vi "Event Handler.vi"(8 "error in (no error)":errorcluster, 10 "Stop Event Handler":refnum<user-event>, 11 "D_Datagrid in":refnum<class "D_Datagrid.lvclass">) -> (0 "error out":errorcluster)   [LabVIEW 2023, in "D Datagrid Library.lvlib" / "D_Datagrid.lvclass"]
doc: "The <b>Event Handler VI</b> is a dynamic dispatch VI that should be overwritten if events are needed to create the enhanced QControl. \n\nBy inheriting from the main Control.lvclass the overwritten <b>Event Handler VI</b> will be launched asynchronously in the initialization of the QControl.\n<b> </b> <b> </b>\n©2016 Q Software Innovations, LLC (QSI)\nwritten by Quentin Alldredge\nproduced in LabVIEW 2015\n\nsupport@qsoftwareinnovations.com\nwww.qsoftwareinnovations.com\n\nAll rights reserved.\n\nRedistribution and use in source and binary forms, with or without modification, are permitted provided that the following conditions are met:\n\n * Redistributions of source code must retain the above copyright notice, this list of conditions and the following disclaimer.\n * Redistributions in binary form must reproduce the above copyright notice, this list of conditions and the following disclaimer in the documentation and/or other materials provided with the distribution.\n * Neither the name of Q Software Innovations, LLC. nor the names of its contributors may be used to endorse or promote products derived from this software without specific prior written permission.\n\nTHIS SOFTWARE IS PROVIDED BY THE COPYRIGHT HOLDERS AND CONTRIBUTORS \"AS IS\" AND ANY EXPRESS OR IMPLIED WARRANTIES, INCLUDING, BUT NOT LIMITED TO, THE IMPLIED WARRANTIES OF MERCHANTABILITY AND FITNESS FOR A PARTICULAR PURPOSE ARE DISCLAIMED. IN NO EVENT SHALL THE COPYRIGHT OWNER OR CONTRIBUTORS BE LIABLE FOR ANY DIRECT, INDIRECT, INCIDENTAL, SPECIAL, EXEMPLARY, OR CONSEQUENTIAL DAMAGES (INCLUDING, BUT NOT LIMITED TO, PROCUREMENT OF SUBSTITUTE GOODS OR SERVICES; LOSS OF USE, DATA, OR PROFITS; OR BUSINESS INTERRUPTION) HOWEVER CAUSED AND ON ANY THEORY OF LIABILITY, WHETHER IN CONTRACT, STRICT LIABILITY, OR TORT (INCLUDING NEGLIGENCE OR OTHERWISE) ARISING IN ANY WAY OUT OF THE USE OF THIS SOFTWARE, EVEN IF ADVISED OF THE POSSIBILITY OF SUCH DAMAGE."
uses:
  D_Datagrid.lvclass
  <vilib>/Utility/miscctls.llb/LVRowAndColumnTypeDef.ctl
  D_Datagrid.lvclass/D_Datagrid.ctl
  DatagridElement/DatagridElement.lvclass/DatagridElement.ctl
  DatagridElement/Read Enabled state.vi
  Read DataElements.vi
  Write DataElements.vi
  Read Auto update indicator.vi
  Redraw full indicator.vi
  <vilib>/Utility/cursorutil.llb/Set Cursor (Icon Pict).vi
  DatagridElement/DatagridElement.lvclass
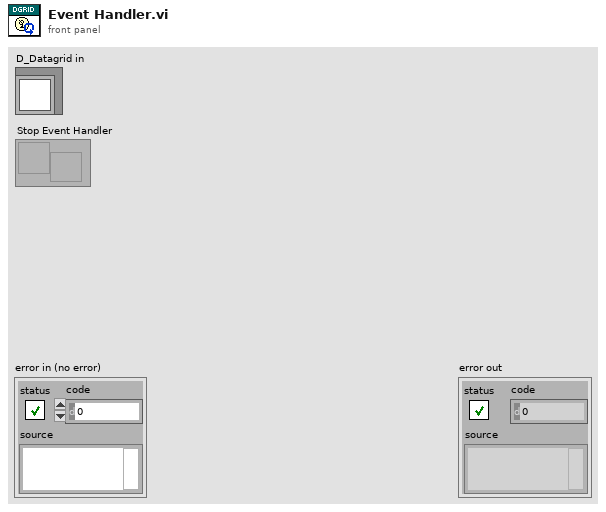
[diagram p1: front panel]
types:
  T1 = typedef "LVRowAndColumnTypeDef.ctl" = cluster{"Row":i32, "Column":i32}
  T2 = typedef "LVPoint32TypeDef.ctl" = cluster{"Horizontal":i32, "Vertical":i32}
  T3 = typedef "LVRectTypeDef.ctl" = cluster{"Left":i16, "Top":i16, "Right":i16, "Bottom":i16}
  T4 = enum8{"Enabled", "Disabled", "Disabled and Grayed Out"}
  T5 = typedef "D Datagrid Library.lvlib/D_Datagrid.lvclass/Scrolling behavior.ctl" = enum16{"Default", "Locked", "Displayed items only"}
  T6 = typedef "LVRowAndColumnUnsignedTypeDef.ctl" = cluster{"Row":u32, "Column":u32}
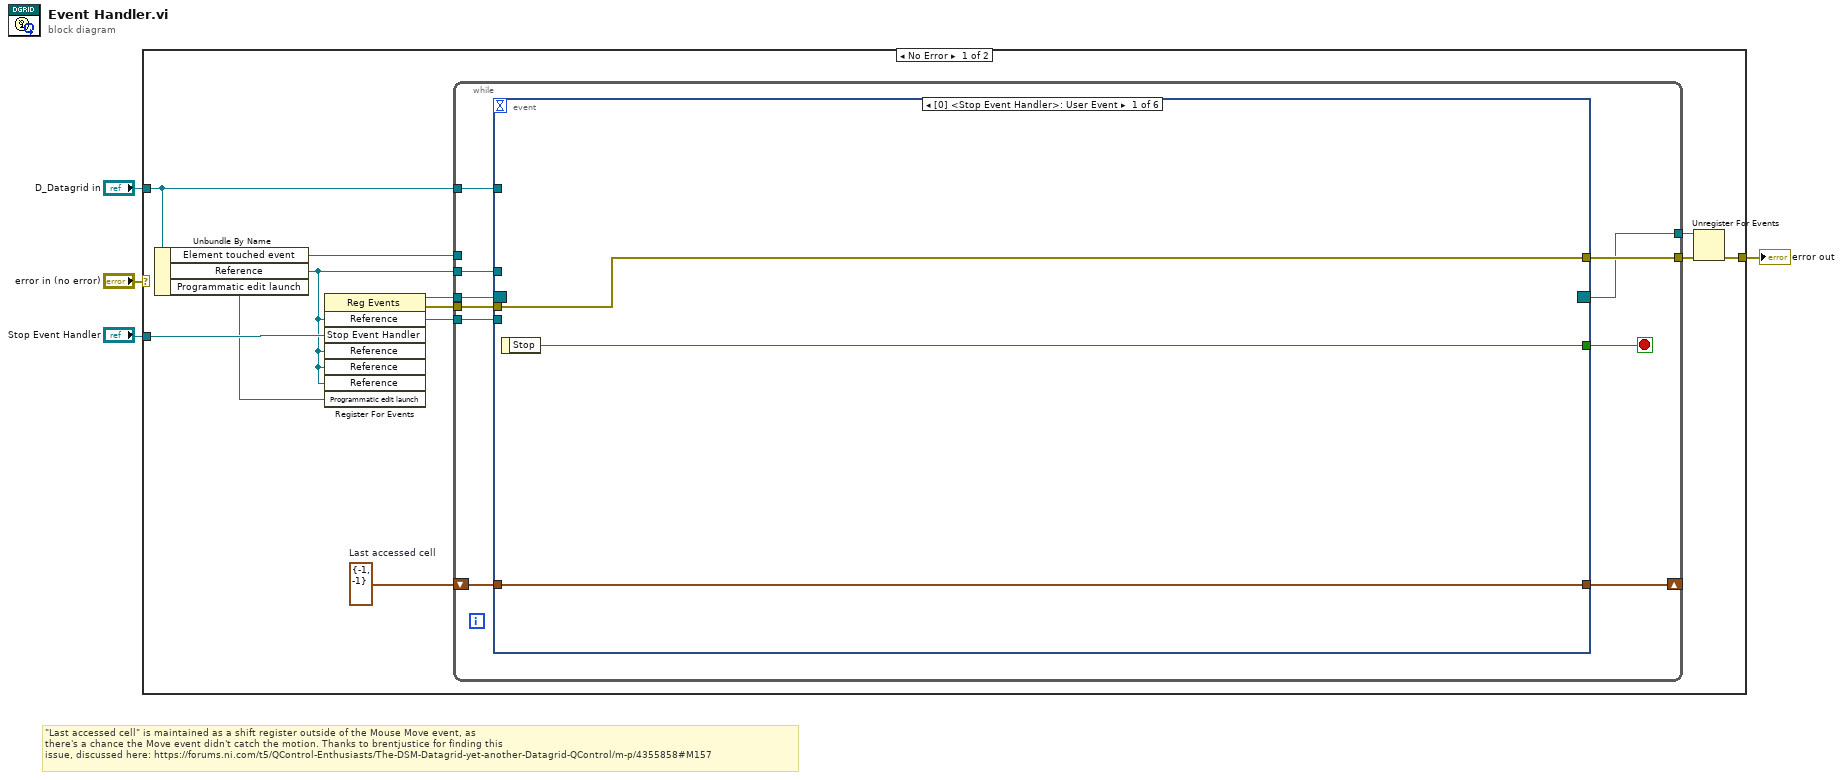
[diagram p0: block diagram]
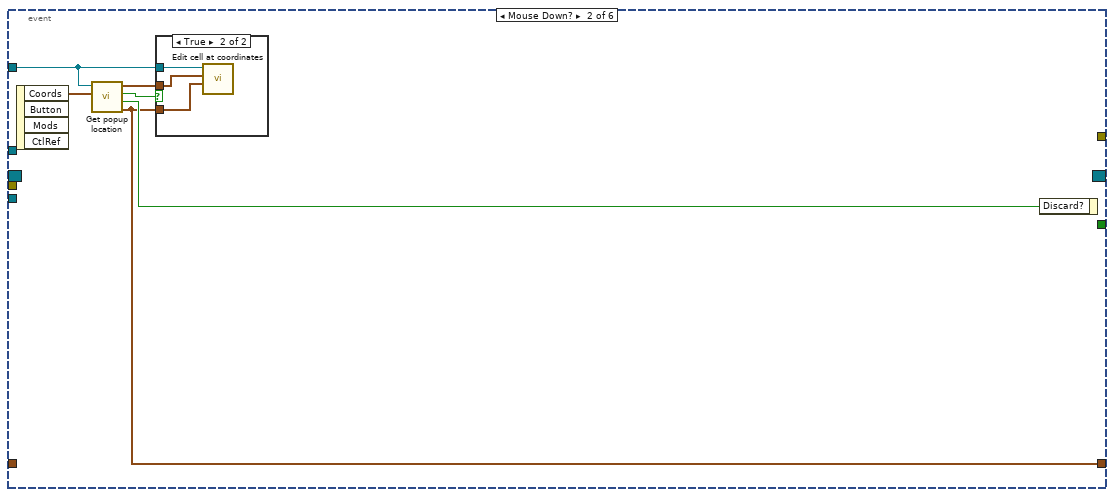
[diagram p2: hidden frame]
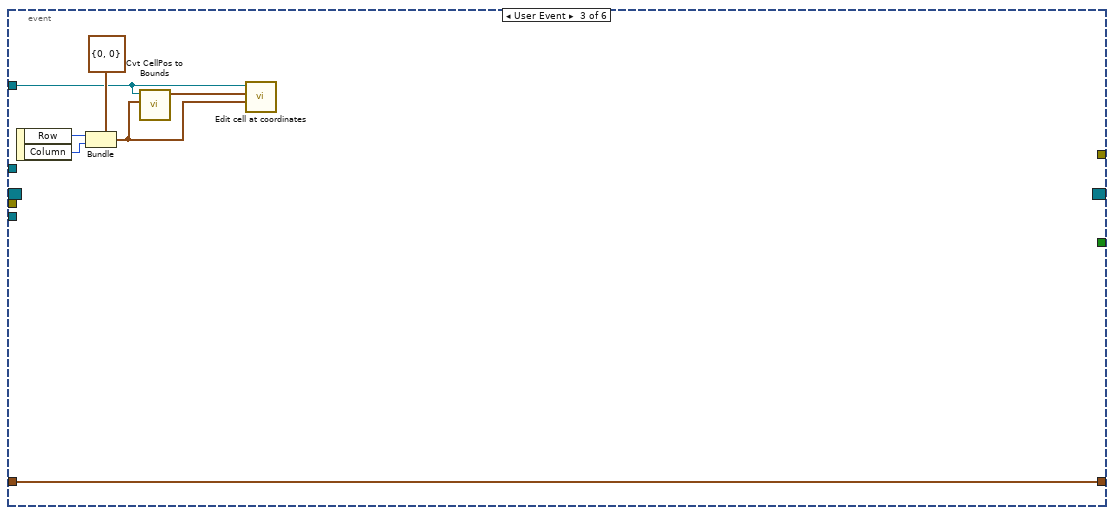
[diagram p4: hidden frame]
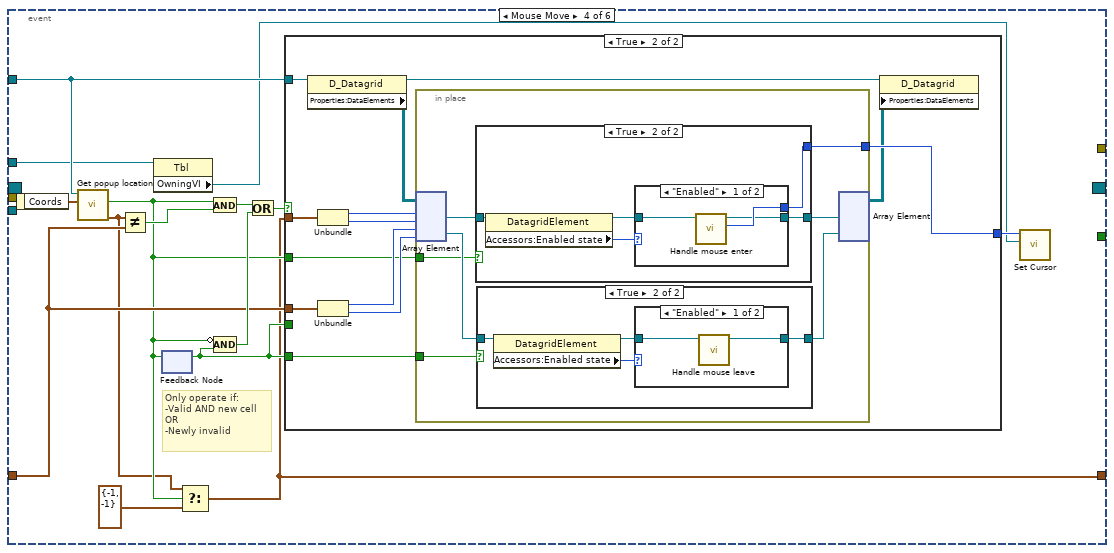
[diagram p5: hidden frame]
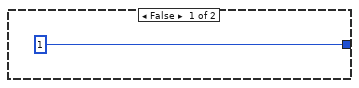
[diagram p6: hidden frame]
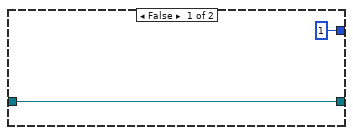
[diagram p9: hidden frame]
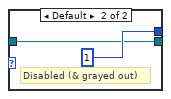
[diagram p10: hidden frame]
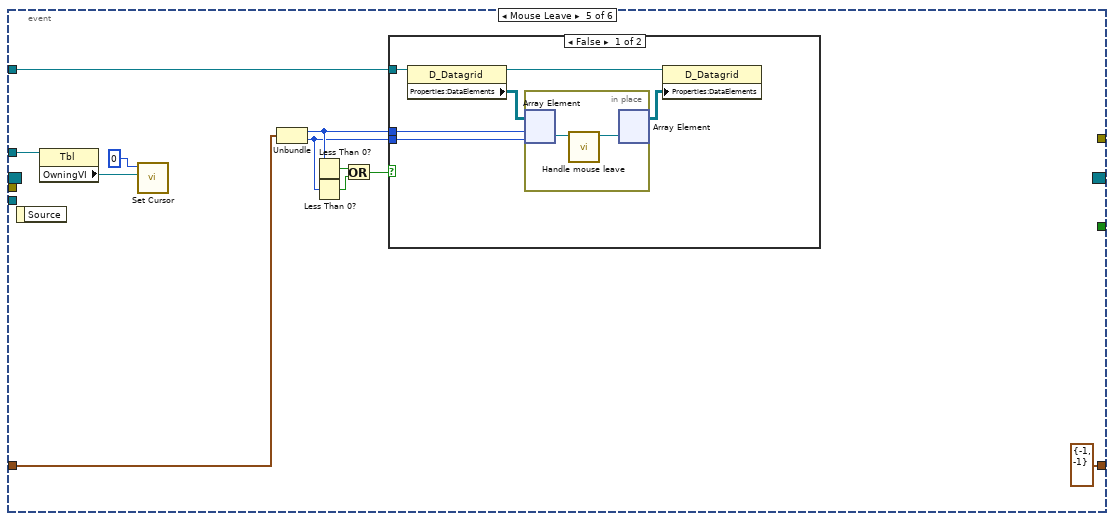
[diagram p11: hidden frame]
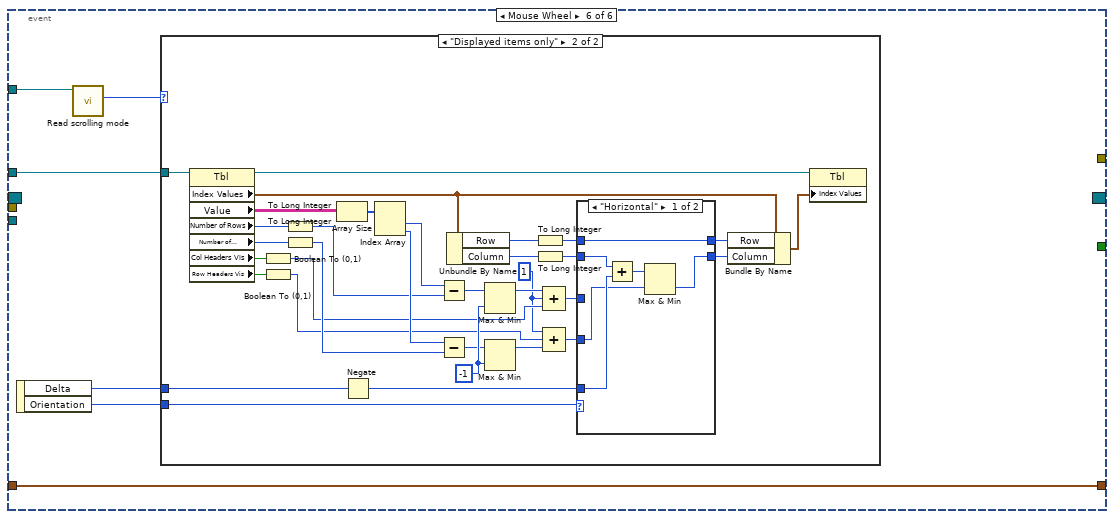
[diagram p13: hidden frame]
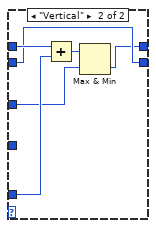
[diagram p15: hidden frame]
diagram:
  # "\"Last accessed cell\" is maintained as a shift register outside of the Mouse Move event, as\nthere's a chance the Move event didn't catch the motion. Thanks to brentjustice for finding this\nissue, discussed here: https://forums.ni.com/t5/QControl-Enthusiasts/The-DSM-Datagrid-yet-another-Datagrid-QControl/m-p/4355858#M157"
  n1 = case shown="No Error" "error in (no error)" {
    selector: "error in (no error)" -> [_ w171]
    tunnel: [w6 w171] -> w3
    tunnel: "D_Datagrid in" -> [w5 _]
    tunnel: "Stop Event Handler" -> [w11 _]
    frame No Error {
      w8 = T1 {"Row"=-1, "Column"=-1}  # Last accessed cell
      n2 = Unbundle By Name(w5) -> ("Element touched event"=w10:refnum<user-event>, "Reference"=w7:refnum<vi>, "Programmatic edit launch"=w9:refnum<user-event>)
      n3 = register-events(w7, w11, w7, w7, w7, w9) -> (reference out=w15:refnum<event-registration>, error out=w14:errorcluster)  [unwired: 2 in]
      n4 = while {
        tunnel: w15 -> [w25]
        tunnel: w14 -> [w23]
        tunnel: [w22] -> w13
        tunnel: [w20] -> w12
        tunnel: w7 -> [w19]
        tunnel: w5 -> [w24]
        tunnel: w7 -> [w18]
        tunnel: w10 -> [_]
        shift-right: [w16] -> _
        shift-left: w8 -> [w17]
        stop <- w21 stop-if-true
        n5 = event shown="[0] <Stop Event Handler>: User Event" {
          selector: w25 -> [_ _ _ _ _ _]
          dyn-events: [_ _ _ _ _ _] -> w20
          timeout: _ -> [_ _ _ _ _ _]
          tunnel: w24 -> [_ w34 w40 w59 w107 w121]
          tunnel: w23 -> [w28 _ _ _ _ _]
          tunnel: [w28 _ _ _ _ _] -> w22
          tunnel: [w27 _ _ _ _ _] -> w21
          tunnel: w19 -> [_ _ _ _ _ _]
          tunnel: w18 -> [_ _ _ w56 w111 w123]
          tunnel: w17 -> [w26 _ w38 w49 w106 w122]
          tunnel: [w26 w29 w38 w45 T1 {"Row"=-1, "Column"=-1} ("Cell Position") w122] -> w16
          event User Event {
            n6 = event-data() -> ("Stop"=w27:bool)  [unwired: 1 in]
          }
          event Mouse Down? {
            n7 = event-data() -> ("Coords"=w32:T2)  [unwired: 1 in, 3 out]
            n8 = call "Get popup location.vi"("Point32"=w32, "D_Datagrid in"=w34) -> ("Cell Position"=w29:T1, "In bounds?"=w31:bool, "Valid cell?"=w30:bool, "Bounds"=w33:T3)  [unwired: 6 in]
            n9 = case shown="True" w30 {
              tunnel: w29 -> [_ w35]
              tunnel: w34 -> [_ w37]
              tunnel: w33 -> [_ w36]
              frame False {
              }
              frame True {
                n10 = call "Edit cell at coordinates.vi"("RowAndCollumn"=w35, "Rect"=w36, "D_Datagrid in"=w37) -> ()  [unwired: 9 in]
              }
            }
            n11 = event-data("Discard?"=w31) -> ()  [unwired: 1 in, 1 out]
          }
          event User Event {
            n12 = event-data() -> ("Row"=w43:i32, "Column"=w42:i32)  [unwired: 1 in]
            n13 = Bundle(cluster=T1 {"Row"=0, "Column"=0} ("CellPosition"), "Row"=w43, "Column"=w42) -> (w39:T1)
            n14 = call "Cvt CellPos to Bounds.vi"("CellPosition"=w39, "D_Datagrid in"=w40) -> ("Bounds"=w41:T3)  [unwired: 9 in]
            n15 = call "Edit cell at coordinates.vi"("RowAndCollumn"=w39, "Rect"=w41, "D_Datagrid in"=w40) -> ()  [unwired: 9 in]
          }
          event Mouse Move {
            # "Only operate if:\n-Valid AND new cell\nOR\n-Newly invalid"
            n16 = event-data() -> ("Coords"=w58:T2)  [unwired: 1 in]
            n17 = call "Get popup location.vi"("Point32"=w58, "D_Datagrid in"=w59) -> ("Cell Position"=w46:T1, "Valid cell?"=w48:bool)  [unwired: 6 in, 2 out]
            n18 = Not Equal?(x=w46, y=w49) -> (x != y?=w54:bool)
            n19 = property class="Tbl"(reference=w56) -> ("OwningVI"=w55:refnum<vi>)  [unwired: 1 in, 2 out]
            n20 = feedback #1() -> (w50:bool)  [unwired: 1 in]
            n21 = feedback-in #1(w48) -> ()
            n22 = Select(t=w46, s=w48, f=T1 {"Row"=-1, "Column"=-1} ("Last accessed cell")) -> (s? t:f=w45:T1)
            n23 = And(x=w48, y=w54) -> (x .and. y?=w53:bool)
            n24 = Compound Arithmetic op=AND(invert w48, w50) -> (w52:bool)
            n25 = Or(x=w53, y=w52) -> (x .or. y?=w51:bool)
            n26 = case shown="True" w51 {
              tunnel: w45 -> [_ w72]
              tunnel: w59 -> [_ w73]
              tunnel: [u16 1 ("Active cursor") w71] -> w57
              tunnel: w49 -> [_ w65]
              tunnel: w48 -> [_ w62]
              tunnel: w50 -> [_ _]
              tunnel: w50 -> [_ w61]
              frame False {
              }
              frame True {
                n27 = property class="D_Datagrid"(reference=w73) -> (reference out=w68:refnum<class "D_Datagrid.lvclass">, "Properties:DataElements"=w66:refnum<class "DatagridElement.lvclass">[][])  [unwired: 1 in, 1 out]
                n28 = Unbundle(w72) -> ("Row"=w70:i32, "Column"=w69:i32)
                n29 = Unbundle(w65) -> ("Row"=w64:i32, "Column"=w63:i32)
                n30 = in-place {
                  in-place-border: [w80] -> w71
                  in-place-border: w62 -> [w75]
                  in-place-border: w61 -> [w74]
                  n31 = in-place-array #2(w66, w70, w69, w64, w63) -> (w79:refnum<class "DatagridElement.lvclass">, w77:refnum<class "DatagridElement.lvclass">)
                  n32 = case shown="True" w75 {
                    tunnel: [u16 1 ("Active cursor") w93] -> w80
                    tunnel: w79 -> [w90 w92]
                    tunnel: [w90 w91] -> w78
                    frame False {
                    }
                    frame True {
                      n33 = property class="DatagridElement"(reference=w92) -> (reference out=w94:refnum<class "DatagridElement.lvclass">, "Accessors:Enabled state"=w95:T4)  [unwired: 1 in, 1 out]
                      n34 = case shown="\"Enabled\"" w95 {
                        tunnel: w94 -> [w98 w99]
                        tunnel: [w97 u16 1 ("Active cursor")] -> w93
                        tunnel: [w96 w99] -> w91
                        frame "Enabled" {
                          n35 = call-dynamic "Handle mouse enter.vi"("DatagridElement in"=w98) -> ("Active cursor"=w97:u16, "DatagridElement out"=w96:refnum<class "DatagridElement.lvclass">)  [unwired: 8 in, 1 out]
                        }
                        frame Default {
                          # "Disabled (& grayed out)"
                        }
                      }
                    }
                  }
                  n36 = case shown="True" w74 {
                    tunnel: w77 -> [w81 w85]
                    tunnel: [w81 w82] -> w76
                    frame False {
                    }
                    frame True {
                      n37 = property class="DatagridElement"(reference=w85) -> (reference out=w83:refnum<class "DatagridElement.lvclass">, "Accessors:Enabled state"=w84:T4)  [unwired: 1 in, 1 out]
                      n38 = case shown="\"Enabled\"" w84 {
                        tunnel: w83 -> [w87 w88]
                        tunnel: [w86 w88] -> w82
                        frame "Enabled" {
                          n39 = call-dynamic "Handle mouse leave.vi"("DatagridElement in"=w87) -> ("DatagridElement out"=w86:refnum<class "DatagridElement.lvclass">)  [unwired: 9 in, 1 out]
                        }
                        frame Default {
                          # "Disabled (& grayed out)"
                        }
                      }
                    }
                  }
                  n40 = in-place-array #2(w78, w76) -> (w67:refnum<class "DatagridElement.lvclass">[][])  [unwired: 4 out]
                }
                n41 = property class="D_Datagrid"(reference=w68, "Properties:DataElements"=w67) -> ()  [unwired: 1 in, 2 out]
              }
            }
            n42 = call-poly <vilib>:"Set Cursor.vi"("VI reference (current VI)"=w55, "icon"=w57) -> ()  [unwired: 8 in, 2 out]
          }
          event Mouse Leave {
            n43 = event-data() -> ()  [unwired: 1 in, 1 out]
            n44 = property class="Tbl"(reference=w111) -> ("OwningVI"=w110:refnum<vi>)  [unwired: 1 in, 2 out]
            n45 = call-poly <vilib>:"Set Cursor.vi"("VI reference (current VI)"=w110, "icon"=u16 0) -> ()  [unwired: 8 in, 2 out]
            n46 = Unbundle(w106) -> ("Row"=w105:i32, "Column"=w104:i32)
            n47 = Less Than 0?(x=w105) -> (x < 0?=w103:bool)
            n48 = Less Than 0?(x=w104) -> (x < 0?=w102:bool)
            n49 = Or(x=w103, y=w102) -> (x .or. y?=w101:bool)
            n50 = case shown="False" w101 {
              tunnel: w107 -> [w114 _]
              tunnel: w105 -> [w113 _]
              tunnel: w104 -> [w112 _]
              frame False {
                n51 = property class="D_Datagrid"(reference=w114) -> (reference out=w117:refnum<class "D_Datagrid.lvclass">, "Properties:DataElements"=w115:refnum<class "DatagridElement.lvclass">[][])  [unwired: 1 in, 1 out]
                n52 = in-place {
                  n53 = in-place-array #3(w115, w113, w112) -> (w119:refnum<class "DatagridElement.lvclass">)
                  n54 = call-dynamic "Handle mouse leave.vi"("DatagridElement in"=w119) -> ("DatagridElement out"=w118:refnum<class "DatagridElement.lvclass">)  [unwired: 9 in, 1 out]
                  n55 = in-place-array #3(w118) -> (w116:refnum<class "DatagridElement.lvclass">[][])  [unwired: 2 out]
                }
                n56 = property class="D_Datagrid"(reference=w117, "Properties:DataElements"=w116) -> ()  [unwired: 1 in, 2 out]
              }
              frame True {
              }
            }
          }
          event Mouse Wheel {
            n57 = event-data() -> ("Delta"=w125:i32, "Orientation"=w124:enum16{"Horizontal", "Vertical"})  [unwired: 1 in]
            n58 = call "Read scrolling mode.vi"("D_Datagrid in"=w121) -> ("Scrolling mode"=w120:T5)  [unwired: 8 in, 2 out]
            n59 = case shown="\"Displayed items only\"" w120 {
              tunnel: w125 -> [_ w137]
              tunnel: w124 -> [_ w136]
              tunnel: w123 -> [_ w158]
              frame "Default", "Locked" {
                # "If default, then LabVIEW handles the scroll wheel.\nIf Locked, LabVIEW doesn't handle it, so don't handle it here either."
              }
              frame "Displayed items only" {
                w126 = i16 1 ("value")
                w155 = -1 ("y")
                n60 = property on="Property Node" class="Tbl"(reference=w158) -> (reference out=w157:refnum<vi>, "Index Values"=w141:T6, "Value"=w140:string[][], "Number of Rows"=w139:u32, "Number of Columns"=w138:u32, "Col Headers Vis"=w130:bool, "Row Headers Vis"=w128:bool)  [unwired: 1 in, 1 out]
                n61 = Boolean To (0,1)(Boolean=w130) -> (0, 1=w129:i16)
                n62 = Boolean To (0,1)(Boolean=w128) -> (0, 1=w127:i16)
                n63 = To Long Integer(number=w139) -> (32bit integer=w150:i32)
                n64 = To Long Integer(number=w138) -> (32bit integer=w152:i32)
                n65 = Array Size(array=w140) -> (size(s)=w142:i32[])
                n66 = Negate(x=w137) -> (-x=w156:i32)
                n67 = Index Array(array=w142) -> (element #1=w149:i32, element #2=w151:i32)  [unwired: 2 in]
                n68 = Subtract(x=w149, y=w150) -> (x-y=w153:i32)
                n69 = Subtract(x=w151, y=w152) -> (x-y=w154:i32)
                n70 = Unbundle By Name(w141) -> ("Row"=w145:u32, "Column"=w146:u32)
                n71 = Max & Min(x=w153, y=w155) -> (max(x,y)=w134:i32)  [unwired: 1 out]
                n72 = Max & Min(x=w154, y=w155) -> (max(x,y)=w132:i32)  [unwired: 1 out]
                n73 = To Long Integer(number=w145) -> (32bit integer=w147:i32)
                n74 = To Long Integer(number=w146) -> (32bit integer=w148:i32)
                n75 = Compound Arithmetic op=ADD(w134, w126, w129) -> (w133:i32)
                n76 = Compound Arithmetic op=ADD(w126, w127, w132) -> (w131:i32)
                n77 = case shown="\"Horizontal\"" w136 {
                  tunnel: [w161 w165] -> w143
                  tunnel: w147 -> [w161 w169]
                  tunnel: w148 -> [w163 w168]
                  tunnel: [w162 w168] -> w144
                  tunnel: w156 -> [w160 w170]
                  tunnel: w133 -> [_ w166]
                  tunnel: w131 -> [w159 _]
                  frame "Horizontal" {
                    n78 = Add(x=w163, y=w160) -> (x+y=w164:i32)
                    n79 = Max & Min(x=w164, y=w159) -> (min(x,y)=w162:i32)  [unwired: 1 out]
                  }
                  frame "Vertical" {
                    n80 = Add(x=w169, y=w170) -> (x+y=w167:i32)
                    n81 = Max & Min(x=w167, y=w166) -> (min(x,y)=w165:i32)  [unwired: 1 out]
                  }
                }
                n82 = Bundle By Name(cluster=w141, "Row"=w143, "Column"=w144) -> (w135:T6)
                n83 = property on="Property Node" class="Tbl"(reference=w157, "Index Values"=w135) -> ()  [unwired: 1 in, 2 out]
              }
            }
          }
        }
      }
      n84 = Unregister For Events(event registration refnum=w12, error in=w13) -> (error out=w6:errorcluster)
    }
    frame Error {
    }
  }
  "error out" <- w3
